vi "SaveSampleData.vi"(6 "采样区域":string, 9 "采样时间":string, 10 "采样数据":string[][](array[string]), 11 "MulticolumnListbox输入":refnum<vi>) -> (3 "保存数据路径":path)   [LabVIEW 2014, in "Sample.lvlib"]
uses:
  <vilib>/Utility/file.llb/Write To Spreadsheet File (string).vi
  Sample/Sample.lvlib
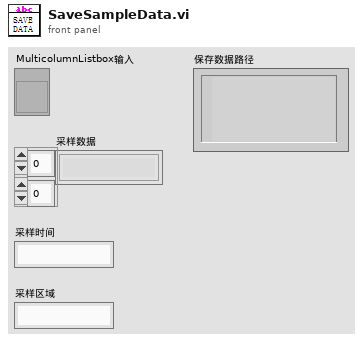
[diagram p1: front panel]
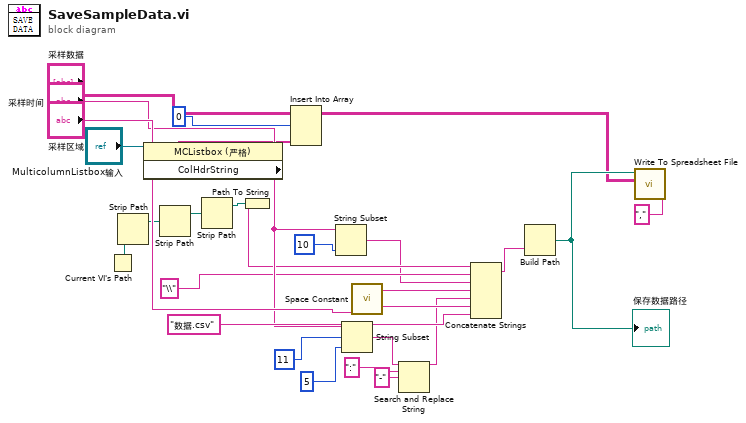
[diagram p0: block diagram]
diagram:
  n1 = Current VI's Path() -> (path=w24:path)
  n2 = Strip Path(path=w24) -> (stripped path=w19:path)  [unwired: 1 out]
  n3 = property on="属性节点" class="MCListbox (严格)"(reference="MulticolumnListbox输入") -> ("ColHdrString"=w3:string[])  [unwired: 1 in, 2 out]
  n4 = Strip Path(path=w19) -> (stripped path=w17:path)  [unwired: 1 out]
  n5 = Strip Path(path=w17) -> (stripped path=w16:path)  [unwired: 1 out]
  n6 = Path To String(path=w16) -> (string=w15:string)
  n7 = Insert Into Array(array="采样数据", index (row)=0, new element=w3) -> (w22:string[][])  [unwired: 1 in]
  n8 = String Subset(string="采样时间", length (rest)=10 ("长度（剩余）")) -> (substring=w7:string)  [unwired: 1 in]
  n9 = String Subset(string="采样时间", offset (0)=11, length (rest)=5) -> (substring=w10:string)
  n10 = call <vilib>:"Space Constant.vi"() -> ("String"=w5:string)
  n11 = Search and Replace String(input string=w10, search string=":" ("搜索字符串"), replace string="-" ("替换字符串(\"\")")) -> (result string=w6:string)  [unwired: 5 in, 3 out]
  n12 = Concatenate Strings(w15, "\\", w7, w5, w6, "采样区域", "数据.csv") -> (w14:string)
  n13 = Build Path(name or relative path=w14) -> (appended path=w23:path)  [unwired: 1 in]
  "保存数据路径" <- w23
  n14 = call-poly <vilib>:"Write To Spreadsheet File.vi"("delimiter (\\t)"="," ("delimiter (\\t)"), "2D data"=w22, "file path (dialog if empty)"=w23) -> ()  [unwired: 5 in, 1 out]
